vi "setStop_Trigger.vi"(8 "error in (no error)":errorcluster, 10 "stop_Trigger":string, 11 "DigitalDevice.lvclass in":refnum<class "DigitalDevice.lvclass">) -> (0 "error out":errorcluster, 3 "DigitalDevice.lvclass out":refnum<class "DigitalDevice.lvclass">)   [LabVIEW 2009, in "Tools.lvlib" / "DatabaseHelpers.lvlib" / "DigitalDevice.lvclass"]
uses:
  DigitalDevice.lvclass
  DigitalDevice.lvclass/DigitalDevice.ctl
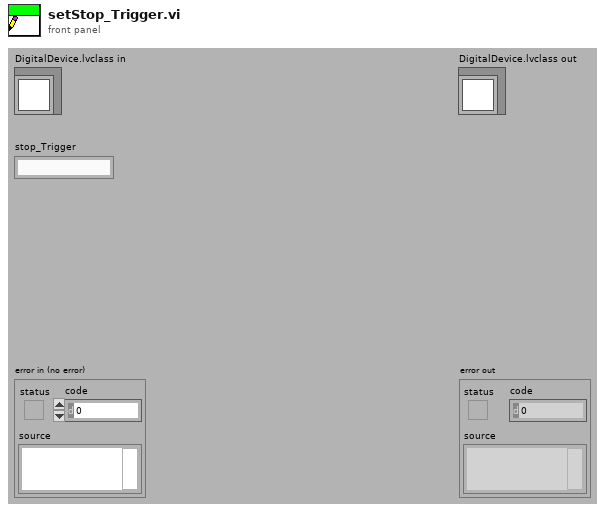
[diagram p1: front panel]
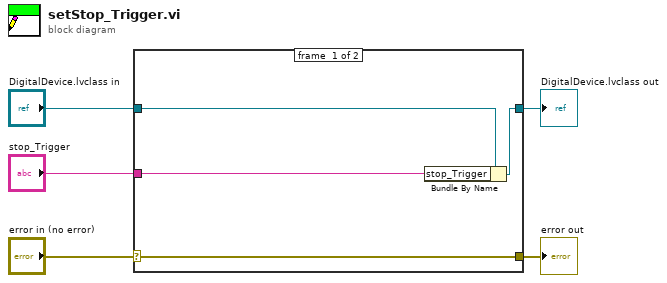
[diagram p0: block diagram]
diagram:
  n1 = case shown="No Error" "error in (no error)" {
    selector: "error in (no error)" -> [w9 w10]
    tunnel: [w9 w10] -> w4
    tunnel: [w7 w11] -> w2
    tunnel: "DigitalDevice.lvclass in" -> [w8 w11]
    tunnel: "stop_Trigger" -> [w6 _]
    frame #0 {
      n2 = Bundle By Name(cluster=w8, "stop_Trigger"=w6) -> (w7:refnum<class "DigitalDevice.lvclass">)
    }
    frame #1 {
    }
  }
  "error out" <- w4
  "DigitalDevice.lvclass out" <- w2
